vi "ArtNet-merger_main.vi"() -> ()   [LabVIEW 2024]
panel:
  out "Waveform Chart":dbl(graph)=2.0
  in  "stop":bool
  in  "get IPs":bool
  in  "IPs":string[](array[string])=["192.168.1.119", "192.168.1.224", "192.168.1.123", "192.168.1.136", "192.168.1.228", "192.168.1.100", "192.168.1.249", "192.168.1.138", "192.168.1.177", "192.168.1.207", "192.168.2.1", "192.168.1.174", "192.168.1.137", "192.168.2.1", "192.168.2.1", "192.168.2.1", "192.168.2.1", "192.168.2.1", "192.168.2.1", "192.168.2.1", "192.168.2.1", "192.168.2.1", "192.168.2.1", "192.168.2.1", "192.168.2.1", "192.168.2.1", "192.168.2.1", "192.168.1.158", "192.168.1.218", "192.168.1.148"]
  in  "Trigger":bool[](array[boolean])=[TRUE, TRUE, TRUE, TRUE, TRUE, TRUE, TRUE, TRUE, TRUE, TRUE, TRUE, TRUE, TRUE, TRUE, TRUE, TRUE, TRUE, TRUE, TRUE, TRUE, TRUE, TRUE, TRUE, TRUE, TRUE, TRUE, TRUE, TRUE, TRUE]
  out "packets per second":dbl=2.0
  in  "Douts":u16[](array[numeric]) caption="dimmer output universe"
  in  "Dchans":u16[](array[numeric]) caption="dimmer channel"
  in  "dimmer input universe":u16=9999
  in  "Output Universes":u16[](array[numeric])=[201, 202, 203, 204, 205, 206, 207, 208, 209, 210, 211, 212, 213, 214, 215, 216, 217, 218, 219, 220, 221, 222, 223, 224, 231, 236, 227, 1, 1, 1]
  in  "Input Patch":u16[](array[numeric])=[201, 202, 203, 204, 205, 206, 207, 208, 209, 210, 211, 212, 213, 214, 215, 216, 217, 218, 219, 220, 221, 222, 223, 224, 231, 227, 236, 11, 1001]
  in  "Output Patch":u16[](array[numeric])=[201, 202, 203, 204, 205, 206, 207, 208, 209, 210, 211, 212, 213, 214, 215, 216, 217, 218, 219, 220, 221, 222, 223, 224, 231, 227, 236, 1, 1]
  in  "Hostnames":string[](array[string])=["wled-LF-LED-Tube-01", "wled-LF-LED-Tube-02", "wled-LF-LED-Tube-03", "wled-LF-LED-Tube-04", "wled-LF-LED-Tube-05", "wled-LF-LED-Tube-06", "wled-LF-LED-Tube-07", "wled-LF-LED-Tube-08", "wled-LF-LED-Tube-09", "wled-LED10", "wled-LF-LED-Tube-11", "wled-LF-LED-Tube-12", "wled-LF-LED-Tube-13", "wled-LF-LED-Tube-14", "wled-LF-LED-Tube-15", "wled-LF-LED-Tube-16", "wled-LF-LED-Tube-17", "wled-LF-LED-Tube-18", "wled-LF-LED-Tube-19", "wled-LF-LED-Tube-20", "wled-LF-LED-Tube-21", "wled-LF-LED-Tube-22", "wled-LF-LED-Tube-23", "wled-LF-LED-Tube-24", "wled-LF-LED-Tube-31", "wled-LF-LED-Tube-36", "wled-LF-LED-Tube-27", "192.168.1.158", "192.168.1.218", "192.168.1.148"]
  in  "stopp":bool
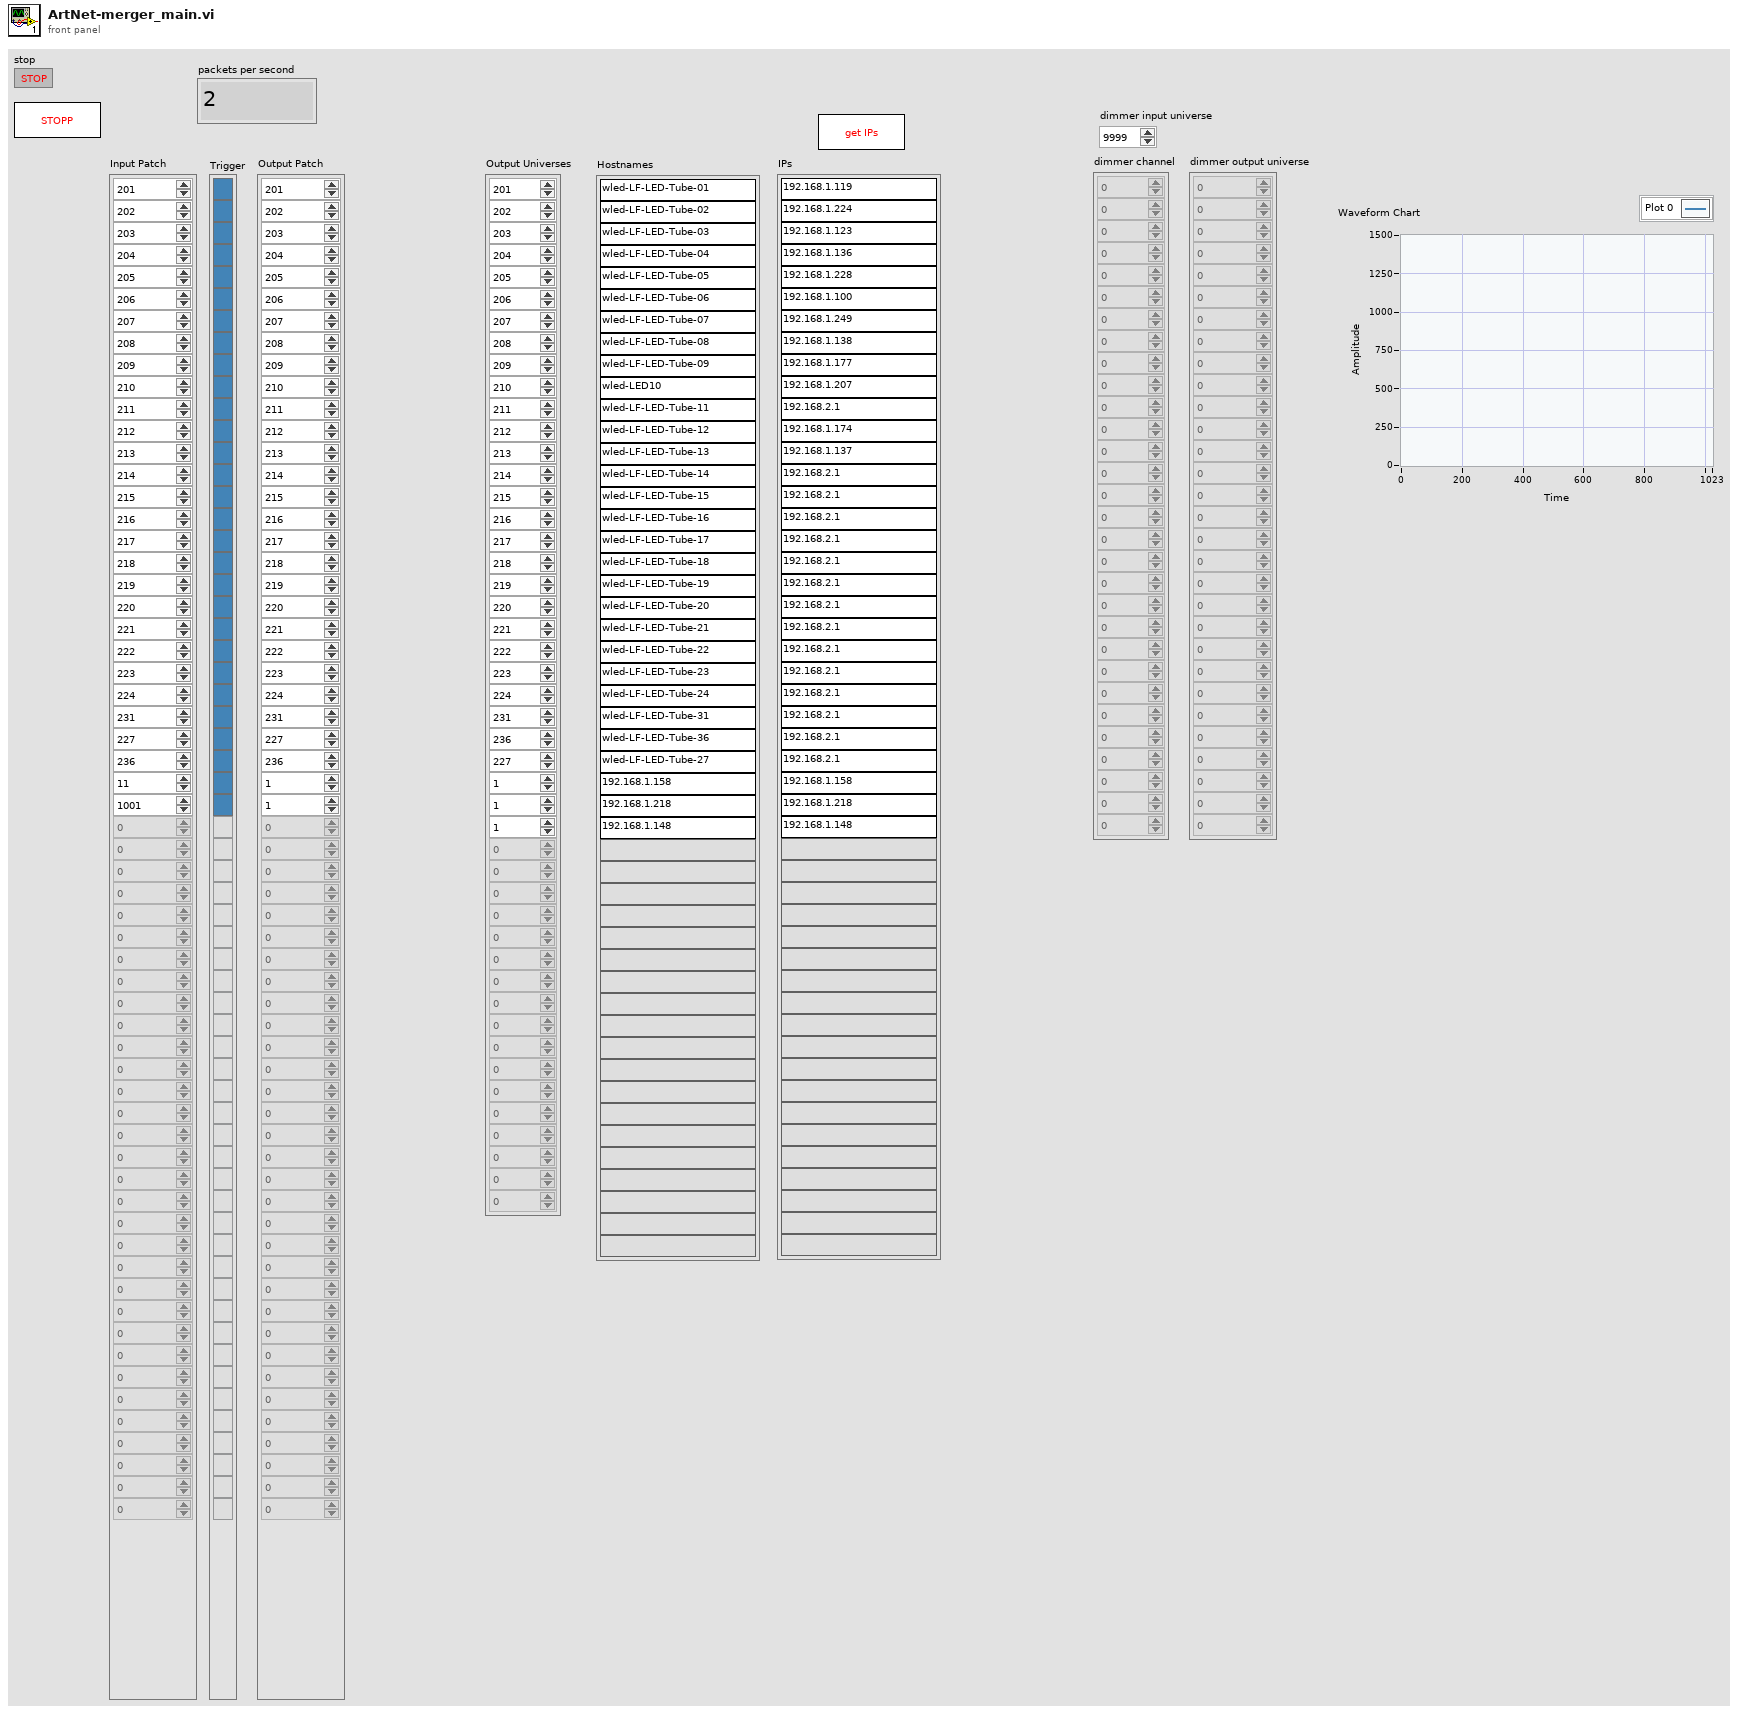
[diagram p1: front panel]
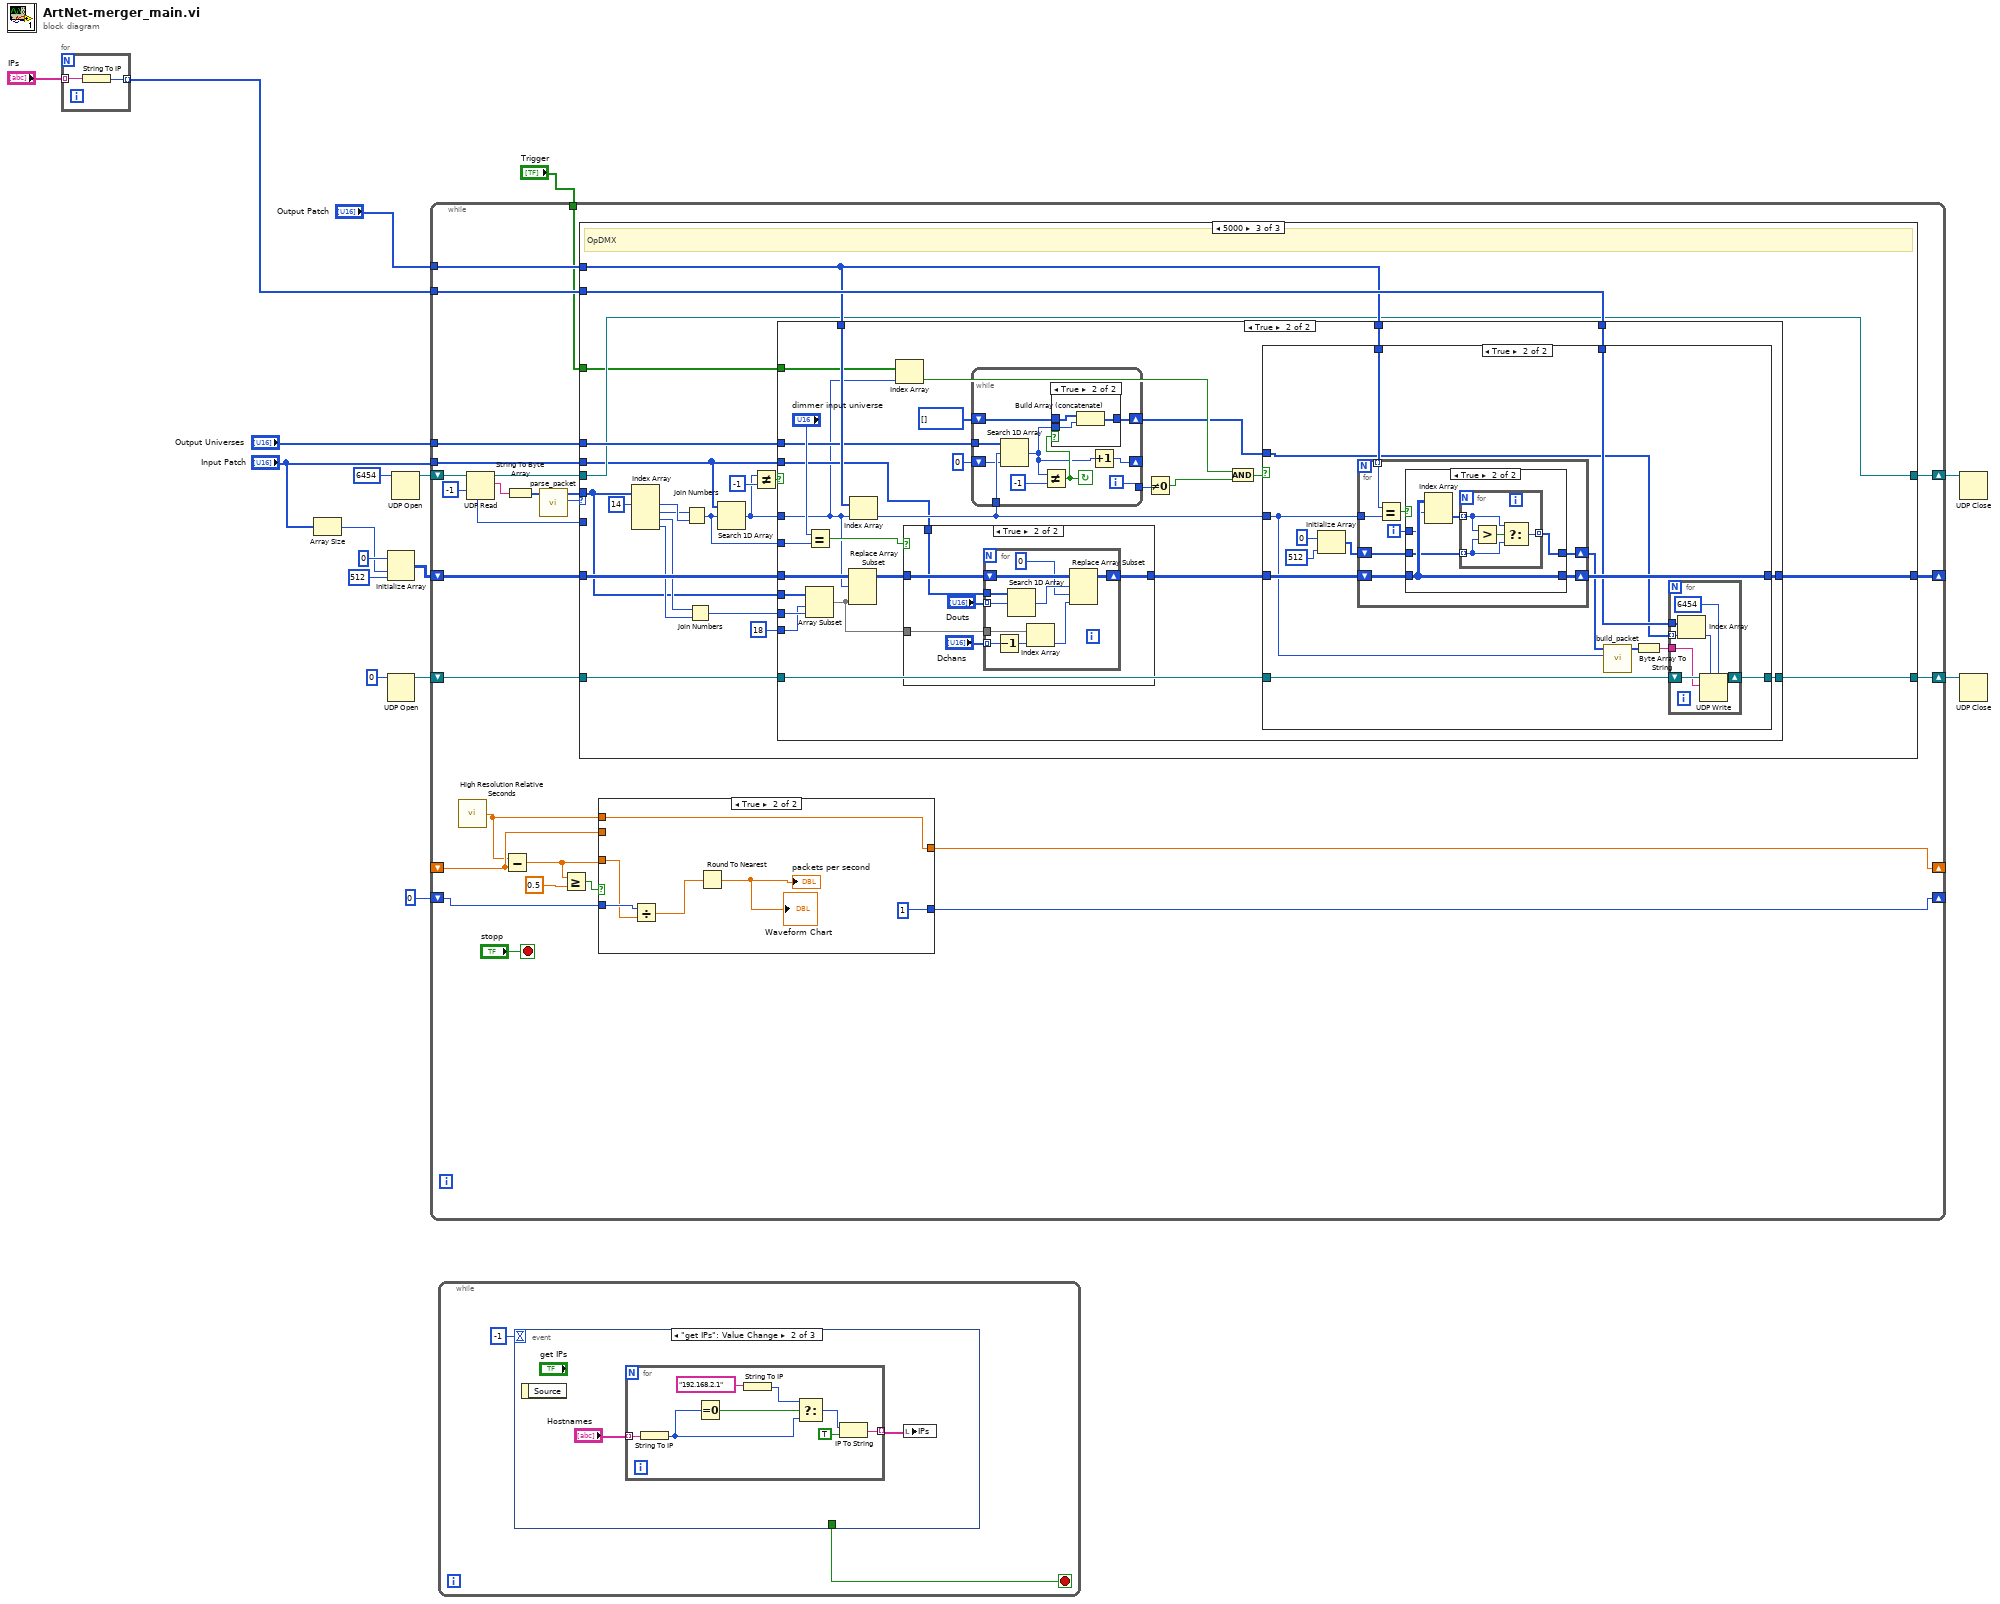
[diagram p0: block diagram]
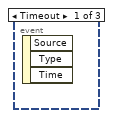
[diagram p2: hidden frame]
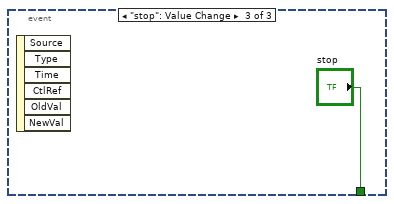
[diagram p3: hidden frame]
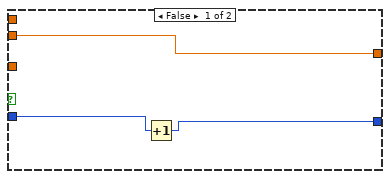
[diagram p4: hidden frame]
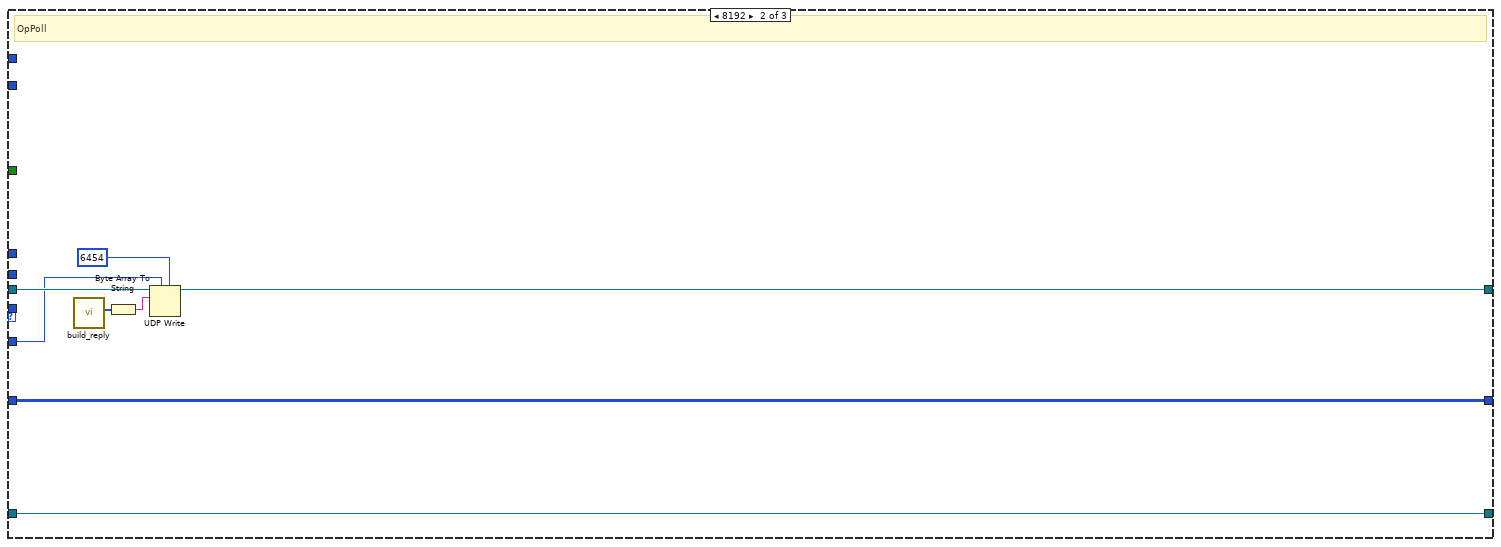
[diagram p6: hidden frame]
diagram:
  n1 = for {
    tunnel: "IPs" -> [w19] mode=indexing
    tunnel: [w18] -> w1 mode=indexing
    n2 = String To IP(1:w19) -> (0:w18:u32)
  }
  n3 = Array Size(array="Input Patch") -> (size(s)=w5:i32)
  n4 = Initialize Array(u8 0, w5, 512 ("dimension size")) -> (w11:u8[][])
  n5 = UDP Open(11:u16 0 ("port")) -> (port=w13:refnum<k16>)  [unwired: 4 in, 2 out]
  n6 = UDP Open(11:u16 6454 ("port")) -> (port=w16:refnum<k16>)  [unwired: 4 in, 2 out]
  n7 = while {
    shift-right: [w30] -> w15
    shift-left: w16 -> [w46]
    tunnel: "Input Patch" -> [w41]
    shift-right: [w40] -> _
    shift-left: w11 -> [w42]
    tunnel: "Output Patch" -> [w36]
    tunnel: "Output Universes" -> [w39]
    tunnel: w1 -> [w38]
    shift-right: [w35] -> w6
    shift-left: w13 -> [w37]
    shift-right: [w22] -> _
    shift-left: _ -> [w23]
    shift-right: [w24] -> _
    shift-left: 0 -> [w25]
    tunnel: "Trigger" -> [w20]
    stop <- "stopp" stop-if-true
    n8 = call <vilib>:"High Resolution Relative Seconds.vi"() -> ("relative seconds"=w21:dbl)
    n9 = UDP Read(connection ID=w46, timeout ms (25000)=-1) -> (data out=w43:string, 3:w31:refnum<k16>, 6:w29:u32)  [unwired: 2 in, 2 out]
    n10 = Subtract(x=w21, y=w23) -> (x-y=w26:dbl)
    n11 = String To Byte Array(string=w43) -> (unsigned byte array=w34:u8[])
    n12 = call "parse_packet.vi"("Packet In"=w34) -> ("op-code"=w33:u16, "Packet Out"=w32:u8[])  [unwired: 9 in]
    n13 = Greater Or Equal?(x=w26, y=0.5) -> (x >= y?=w27:bool)
    n14 = case shown="5000" w33 {
      tunnel: w42 -> [w58 w60 w88]
      tunnel: w41 -> [_ _ w69]
      tunnel: [w58 w60 w87] -> w40
      tunnel: w39 -> [_ _ w86]
      tunnel: w38 -> [_ _ w85]
      tunnel: w37 -> [w57 w59 w84]
      tunnel: w36 -> [_ _ w83]
      tunnel: [w57 w59 w82] -> w35
      tunnel: w32 -> [_ _ w67]
      tunnel: w31 -> [w56 w66 w78]
      tunnel: [w56 w61 w78] -> w30
      tunnel: w29 -> [_ w62 _]
      tunnel: w20 -> [_ _ w68]
      frame 0, Default {
      }
      frame 8192 {
        # "OpPoll"
        n15 = call "build_reply.vi"() -> ("output array"=w65:u8[])  [unwired: 11 in]
        n16 = Byte Array To String(unsigned byte array=w65) -> (string=w64:string)
        n17 = UDP Write(address=w62, port or service name=u16 6454 ("port"), connection ID=w66, data in=w64) -> (3:w61:refnum<k16>)  [unwired: 2 in, 1 out]
      }
      frame 20480 {
        # "OpDMX"
        n18 = Index Array(array=w67, index #1=14 ("index")) -> (element #1=w77:u8, element #2=w76:u8, element #3=w74:u8, element #4=w75:u8)  [unwired: 3 in]
        n19 = Join Numbers ("universe")(hi=w76, lo=w77) -> ((hi.lo)=w70:u16)
        n20 = Join Numbers(hi=w74, lo=w75) -> ((hi.lo)=w72:u16)
        n21 = Search 1D Array(1D array=w69, element=w70) -> (index of element=w79:i32)  [unwired: 1 in]
        n22 = Not Equal?(x=w79, y=-1) -> (x != y?=w80:bool)
        n23 = case shown="True" w80 {
          tunnel: w88 -> [w90 w111]
          tunnel: w79 -> [_ w99]
          tunnel: w86 -> [_ w103]
          tunnel: w85 -> [_ w113]
          tunnel: w84 -> [w89 w118]
          tunnel: w83 -> [_ w117]
          tunnel: [w90 w116] -> w87
          tunnel: w83 -> [_ w114]
          tunnel: [w89 w112] -> w82
          tunnel: w67 -> [_ w110]
          tunnel: w72 -> [_ w109]
          tunnel: 18 ("index") -> [_ w108]
          tunnel: w70 -> [_ w107]
          tunnel: w69 -> [_ w102]
          tunnel: w68 -> [_ w98]
          frame False {
          }
          frame True {
            n24 = Equal?(x="dimmer input universe", y=w107) -> (x = y?=w101:bool)
            n25 = Array Subset(array=w110, index=w108, length=w109) -> (w105:u8[])
            n26 = Replace Array Subset(array=w111, new element=w105, index (row)=w99) -> (w104:u8[][])  [unwired: 1 in]
            n27 = Index Array(array=w117, index=w99) -> (element=w115:u16)
            n28 = Index Array(array=w98, index=w99) -> (element=w97:bool)
            n29 = case shown="True" w101 {
              tunnel: w105 -> [_ w139]
              tunnel: w104 -> [w133 w138]
              tunnel: w102 -> [_ w135]
              tunnel: [w133 w134] -> w100
              frame False {
              }
              frame True {
                n30 = for {
                  tunnel: w139 -> [w149]
                  tunnel: "Douts" -> [w145] mode=indexing
                  tunnel: "Dchans" -> [w147] mode=indexing
                  tunnel: w135 -> [w146]
                  shift-right: [w143] -> w134
                  shift-left: w138 -> [w144]
                  n31 = Decrement(x=w147) -> (x-1=w148:u16)
                  n32 = Search 1D Array(1D array=w146, element=w145) -> (index of element=w142:i32)  [unwired: 1 in]
                  n33 = Index Array(array=w149, index=w148) -> (element=w141:u8)
                  n34 = Replace Array Subset(array=w144, new element=w141, index (row)=w142, index (col)=0 ("disabled index (col)")) -> (w143:u8[][])
                }
              }
            }
            n35 = while {
              tunnel: w115 -> [w128]
              tunnel: w103 -> [w126]
              shift-right: [w120] -> _
              shift-left: 0 ("index of element") -> [w125]
              shift-right: [w123] -> w93
              shift-left: i32[] [] -> [w122]
              tunnel: [w121] -> w92
              i -> [w121]
              stop <- w124 continue-if-true
              n36 = Search 1D Array(1D array=w126, element=w128, start index (0)=w125) -> (index of element=w119:i32)
              n37 = Not Equal?(x=w119, y=-1) -> (x != y?=w124:bool)
              n38 = case shown="True" w124 {
                tunnel: w119 -> [_ w132]
                tunnel: [w129 w131] -> w123
                tunnel: w122 -> [w129 w130]
                frame False {
                }
                frame True {
                  n39 = Build Array (concatenate)(w130, w132) -> (w131:i32[])
                }
              }
              n40 = Increment(x=w119) -> (x+1=w120:i32)
            }
            n41 = Not Equal To 0?(x=w92) -> (x != 0?=w91:bool)
            n42 = And(x=w97, y=w91) -> (x .and. y?=w96:bool)
            n43 = case shown="True" w96 {
              tunnel: w118 -> [w150 w165]
              tunnel: w93 -> [_ w156]
              tunnel: w100 -> [w151 w163]
              tunnel: [w151 w162] -> w116
              tunnel: w115 -> [_ w153]
              tunnel: w114 -> [_ w164]
              tunnel: w113 -> [_ w157]
              tunnel: [w150 w155] -> w112
              frame False {
              }
              frame True {
                n44 = Initialize Array(u8 0, 512 ("dimension size")) -> (w159:u8[])
                n45 = for {
                  tunnel: w153 -> [w178]
                  tunnel: w164 -> [w180] mode=indexing
                  shift-right: [w175] -> w162
                  shift-left: w163 -> [w179]
                  shift-right: [w174] -> w154
                  shift-left: w159 -> [w176]
                  i -> [w173]
                  n46 = Equal?(x=w180, y=w178) -> (x = y?=w177:bool)
                  n47 = case shown="True" w177 {
                    tunnel: w179 -> [w182 w187]
                    tunnel: w176 -> [w181 w186]
                    tunnel: [w182 w187] -> w175
                    tunnel: [w181 w184] -> w174
                    tunnel: w173 -> [_ w183]
                    frame False {
                    }
                    frame True {
                      n48 = Index Array(array=w187, index (row)=w183) -> (element=w185:u8[])  [unwired: 1 in]
                      n49 = for {
                        tunnel: w186 -> [w189] mode=indexing
                        tunnel: w185 -> [w190] mode=indexing
                        tunnel: [w188] -> w184 mode=indexing
                        n50 = Greater?(x=w190, y=w189) -> (0:w191:bool)
                        n51 = Select(t=w190, s=w191, f=w189) -> (s? t:f=w188:u8)
                      }
                    }
                  }
                }
                n52 = call "build_packet.vi"("universe"=w153, "Data In"=w154) -> ("Packet Out"=w152:u8[])  [unwired: 9 in]
                n53 = Byte Array To String(unsigned byte array=w152) -> (string=w158:string)
                n54 = for {
                  tunnel: w158 -> [w170]
                  tunnel: w157 -> [w169]
                  tunnel: w156 -> [w168] mode=indexing
                  shift-right: [w167] -> w155
                  shift-left: w165 -> [w171]
                  n55 = Index Array(array=w169, index=w168) -> (element=w166:u32)
                  n56 = UDP Write(address=w166, port or service name=u16 6454, connection ID=w171, data in=w170) -> (3:w167:refnum<k16>)  [unwired: 2 in, 1 out]
                }
              }
            }
          }
        }
      }
    }
    n57 = case shown="True" w27 {
      tunnel: w26 -> [_ w54]
      tunnel: w25 -> [w48 w55]
      tunnel: [w47 1] -> w24
      tunnel: w23 -> [w49 _]
      tunnel: [w49 w53] -> w22
      tunnel: w21 -> [_ w53]
      frame False {
        n58 = Increment(x=w48) -> (x+1=w47:i32)
      }
      frame True {
        n59 = Divide(x=w55, y=w54) -> (x/y=w51:dbl)
        n60 = Round To Nearest(number=w51) -> (nearest integer value=→"packets per second" →"Waveform Chart":dbl)
      }
    }
  }
  n61 = while {
    stop <- w193 stop-if-true
    n62 = event shown="[1] \"get IPs\": Value Change" {
      selector: _ -> [_ _ _]
      dyn-events: _ -> [_ _ _]
      timeout: -1 -> [_ _ _]
      tunnel: [_ _ "stop"] -> w193
      event Timeout {
        n63 = event-data() -> ()  [unwired: 1 in, 3 out]
      }
      event "get IPs": Value Change {
        n64 = event-data() -> ()  [unwired: 1 in, 1 out]
        n65 = for {
          tunnel: "Hostnames" -> [w203] mode=indexing
          tunnel: [w196] -> w194 mode=indexing
          n66 = String To IP(1:w203) -> (0:w201:u32)
          n67 = Equal To 0?(x=w201) -> (x = 0?=w202:bool)
          n68 = String To IP(1:"192.168.2.1" ("name")) -> (0:w200:u32)
          n69 = Select(t=w200, s=w202, f=w201) -> (s? t:f=w198:u32)
          n70 = IP To String(1:TRUE ("dot notation? (F)"), 2:w198) -> (0:w196:string)
        }
        n71 = local write "IPs"(w194) -> ()
      }
      event "stop": Value Change {
        n72 = event-data() -> ()  [unwired: 1 in, 6 out]
      }
    }
  }
  n73 = UDP Close(connection ID=w15) -> ()  [unwired: 1 in, 2 out]
  n74 = UDP Close(connection ID=w6) -> ()  [unwired: 1 in, 2 out]
